vi "test_Build path.vi"(8 "error in (no error)":errorcluster, 11 "TestCase in":refnum<class "[Test Case] Build path.lvclass">) -> (0 "error out":errorcluster, 3 "TestCase out":refnum<class "[Test Case] Build path.lvclass">)   [LabVIEW 2016, in "Tests.lvlib" / "[Test Case] Build path.lvclass"]
uses:
  [Test Case] Build path.lvclass
  [Test Case] Build path.lvclass/[Test Case] Build path.ctl
  <vilib>/addons/_JKI Toolkits/VI Tester/TestCase.llb/TestCase.lvclass
  classes/File Transfer Behavior/File Transfer Behavior.lvclass
  C:/Program Files (x86)/National Instruments/LabVIEW 2016/vi.lib/addons/_JKI Toolkits/VI Tester/TestCase.llb/TestCase.lvclass
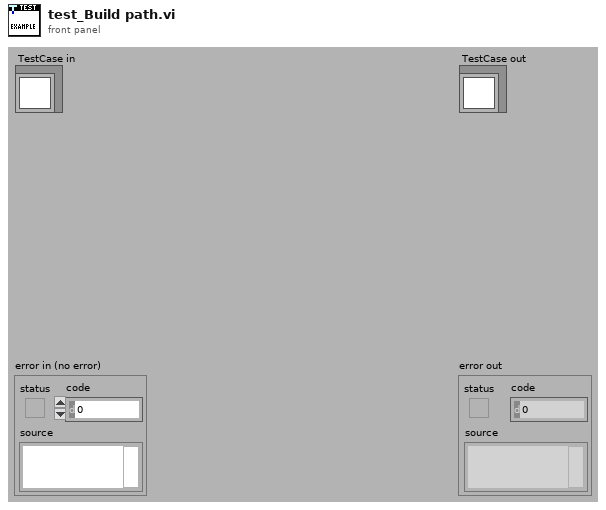
[diagram p1: front panel]
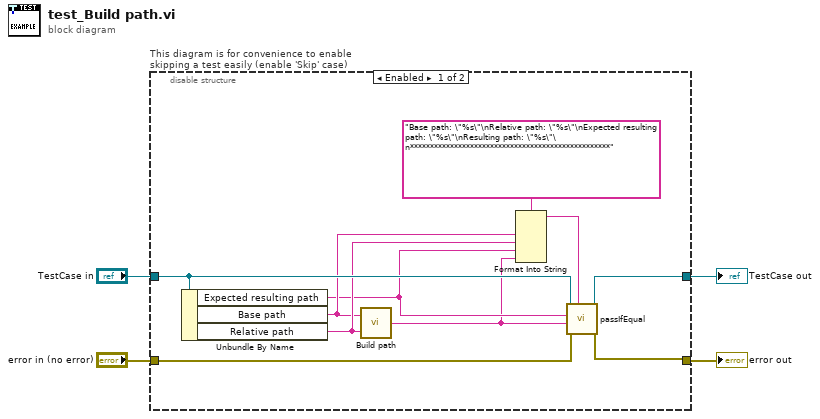
[diagram p0: block diagram]
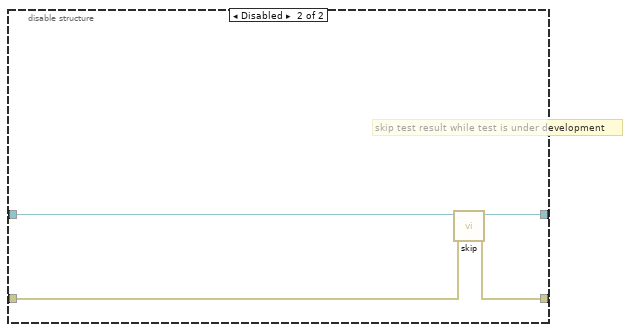
[diagram p2: hidden frame]
diagram:
  n1 = disable-structure "This diagram is for convenience to enable skipping a test easily (enable 'Skip' case)" shown="Enabled" {
    disable-tunnel: "TestCase in" -> [w12 w18]
    disable-tunnel: [w14 w16] -> w1
    disable-tunnel: [w13 w17] -> w3
    disable-tunnel: "error in (no error)" -> [w11 w15]
    frame Enabled {
      n2 = Unbundle By Name(w12) -> ("Expected resulting path"=w6:string, "Base path"=w7:string, "Relative path"=w8:string)
      n3 = call "Build path.vi"("Relative path"=w8, "Base path"=w7) -> ("Resulting path"=w5:string)
      n4 = Format Into String(format string="Base path: \"%s\"\nRelative path: \"%s\"\nExpected resulting path: \"%s\"\nResulting path: \"%s\"\n**************************************************", w7, w8, w6, w5) -> (resulting string=w10:string)  [unwired: 2 in, 1 out]
      n5 = call-dynamic "passIfEqual.vi"("custom report message (\"\")"=w10, "error in (no error)"=w11, "y"=w5, "x"=w6, "TestCase in"=w12) -> ("error out"=w13:errorcluster, "TestCase out"=w14:refnum<class "[Test Case] Build path.lvclass">)  [unwired: 5 in]
    }
    frame Disabled {
      # "skip test result while test is under development"
      n6 = call <vilib>:"skip.vi"("error in (no error)"=w15, "TestCase in"=w18) -> ("error out"=w17:errorcluster, "TestCase out"=w16:refnum<class "[Test Case] Build path.lvclass">)  [unwired: 8 in]
    }
  }
  "error out" <- w3
  "TestCase out" <- w1
